vi "LED_Controller.vi"() -> ()   [LabVIEW 2016]
doc: "Controlls the intention LED strip. There are 4 different light states, startup, idle, navigating, warning.\nStartup - blinking yellow\nIdle - rotating green\nNavigating - directional white/green light\nWarning - rotating red"
uses:
  GlobalVI.vi
  <userlib>/ROS for LabVIEW Software/ROS/Code/_ROSDefinition.vi
panel:
  out "unicornCurrentState":i32
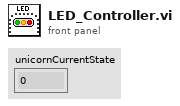
[diagram p1: front panel]
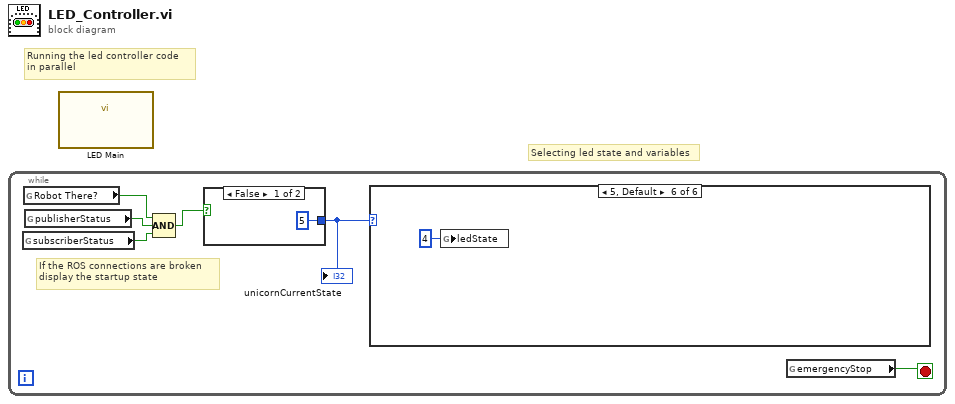
[diagram p0: block diagram]
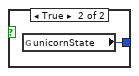
[diagram p2: hidden frame]
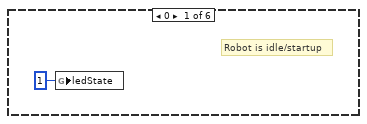
[diagram p3: hidden frame]
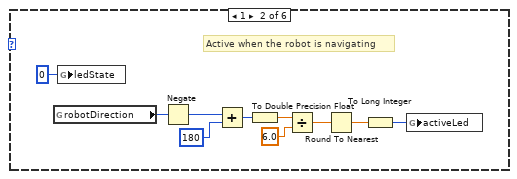
[diagram p4: hidden frame]
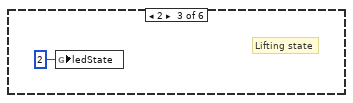
[diagram p5: hidden frame]
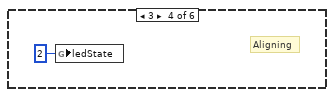
[diagram p6: hidden frame]
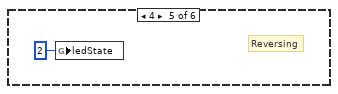
[diagram p7: hidden frame]
diagram:
  # "Selecting led state and variables"
  # "Running the led controller code\nin parallel"
  n1 = while {
    stop <- w6 stop-if-true
    # "If the ROS connections are broken\ndisplay the startup state"
    n2 = global read "GlobalVI.vi" "subscriberStatus"() -> (w5:bool)
    n3 = global read "_ROSDefinition.vi" "Robot There?"() -> (w3:bool)
    n4 = global read "GlobalVI.vi" "publisherStatus"() -> (w4:bool)
    n5 = Compound Arithmetic op=AND(w3, w4, w5) -> (w2:bool)
    n6 = case shown="False" w2 {
      tunnel: [5 ("unicornState") w8] -> w1
      frame False {
      }
      frame True {
        n7 = global read "GlobalVI.vi" "unicornState"() -> (w8:i32)
      }
    }
    "unicornCurrentState" <- w1
    n8 = case shown="5, Default" w1 {
      frame 0 {
        # "Robot is idle/startup"
        n9 = global write "GlobalVI.vi" "ledState"(1 ("ledState")) -> ()
      }
      frame 1 {
        # "Active when the robot is navigating"
        n10 = global read "GlobalVI.vi" "robotDirection"() -> (w11:i32)
        n11 = global write "GlobalVI.vi" "ledState"(0 ("ledState")) -> ()
        n12 = Negate(x=w11) -> (-x=w10:i32)
        n13 = Add(x=w10, y=180) -> (x+y=w17:i32)
        n14 = To Double Precision Float(number=w17) -> (double precision float=w16:dbl)
        n15 = Divide(x=w16, y=6.0) -> (x/y=w14:dbl)
        n16 = Round To Nearest(number=w14) -> (nearest integer value=w13:dbl)
        n17 = To Long Integer(number=w13) -> (32bit integer=w12:i32)
        n18 = global write "GlobalVI.vi" "activeLed"(w12) -> ()
      }
      frame 2 {
        # "Lifting state"
        n19 = global write "GlobalVI.vi" "ledState"(2 ("ledState")) -> ()
      }
      frame 3 {
        # "Aligning"
        n20 = global write "GlobalVI.vi" "ledState"(2 ("ledState")) -> ()
      }
      frame 4 {
        # "Reversing"
        n21 = global write "GlobalVI.vi" "ledState"(2 ("ledState")) -> ()
      }
      frame 5, Default {
        n22 = global write "GlobalVI.vi" "ledState"(4 ("ledState")) -> ()
      }
    }
    n23 = global read "GlobalVI.vi" "emergencyStop"() -> (w6:bool)
  }
  n24 = call "LED Main.vi"() -> ()  [unwired: 11 in]
